vi "replace cursor action stack.vi"(7 "stack action":T2, 8 "action list I":T1[](array[typedef]), 9 "cursor action":T1=enum."write", 11 "command stack In":T1[](array[typedef])) -> (1 "cursor action Out":T1=enum."write", 2 "stack is empty ?":bool, 3 "command stack Out":T1[](array[typedef]))   [LabVIEW 2018]
uses:
  stack action -- control.ctl
  cursor action.ctl
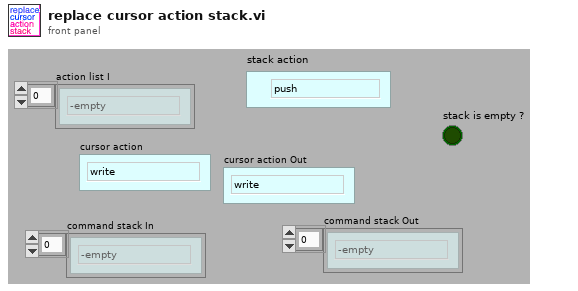
[diagram p1: front panel]
types:
  T1 = typedef "cursor action.ctl" = enum16{"range", "read", "write", "check", "zoom out", "smart zoom out", "zoom to aspect ratio 1", "zoom to win", "zoom out 20%", "zoom in 20%", "-empty", "smart zoom out&aspect", "move range left 20%", "move range right 20%", "move range up 20%", "move range down 20%", "zoom to X win", "zoom to Y win", "zoom out X", "zoom out Y", "zoom in X", "zoom in Y", "check plot scale"}
  T2 = typedef "stack action -- control.ctl" = enum16{"push", "pop", "check", "init"}
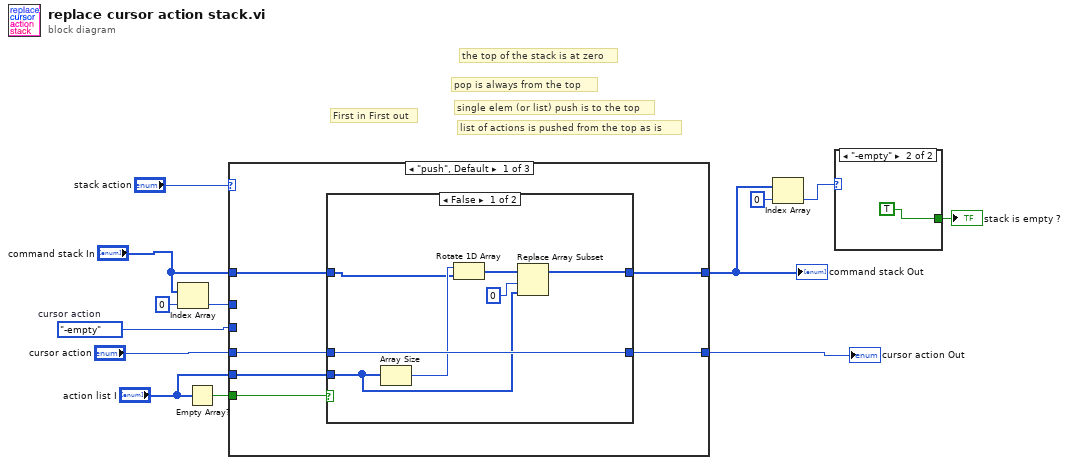
[diagram p0: block diagram]
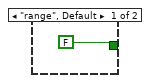
[diagram p2: hidden frame]
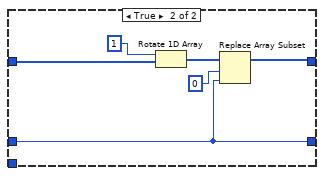
[diagram p3: hidden frame]
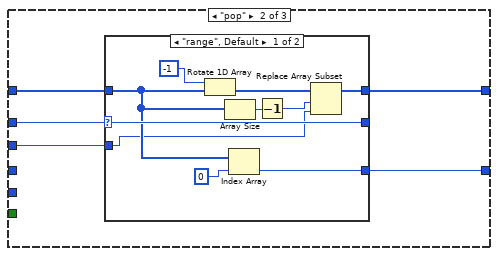
[diagram p4: hidden frame]
diagram:
  w6 = cursor_action."-empty"  # cursor action
  # "list of actions is pushed from the top as is"
  # "single elem (or list) push is to the top"
  # "pop is always from the top"
  # "First in First out"
  # "the top of the stack is at zero"
  n1 = Index Array(array="command stack In", index=0) -> (element=w10:T1)
  n2 = Empty Array?(array="action list I") -> (empty?=w12:bool)
  n3 = case shown="\"push\", Default" "stack action" {
    tunnel: [w19 w37 w51] -> w2
    tunnel: "command stack In" -> [w18 w36 w51]
    tunnel: w10 -> [_ w35 _]
    tunnel: [w14 w34 w52] -> w4
    tunnel: "cursor action" -> [w17 _ w52]
    tunnel: w12 -> [w16 _ _]
    tunnel: "action list I" -> [w15 _ _]
    tunnel: w6 -> [_ w33 _]
    frame "push", Default {
      n4 = case shown="False" w16 {
        tunnel: [w20 w27] -> w19
        tunnel: w18 -> [w24 w29]
        tunnel: w17 -> [w26 w30]
        tunnel: w15 -> [w21 _]
        tunnel: [w26 w30] -> w14
        frame False {
          n5 = Array Size(array=w21) -> (size(s)=w25:i32)
          n6 = Rotate 1D Array(1:w24, 2:w25) -> (0:w23:T1[])
          n7 = Replace Array Subset(array=w23, new element=w21, index=0) -> (w20:T1[])
        }
        frame True {
          n8 = Rotate 1D Array(1:w29, 2:1) -> (0:w32:T1[])
          n9 = Replace Array Subset(array=w32, new element=w30, index=0) -> (w27:T1[])
        }
      }
    }
    frame "pop" {
      n10 = case shown="\"range\", Default" w35 {
        selector: w35 -> [w45 w49]
        tunnel: [w41 w50] -> w37
        tunnel: w36 -> [w42 w50]
        tunnel: [w46 w48] -> w34
        tunnel: [w45 w49] -> _
        tunnel: w33 -> [w38 w48]
        frame "range", Default {
          n11 = Rotate 1D Array(1:w42, 2:-1) -> (0:w40:T1[])
          n12 = Array Size(array=w42) -> (size(s)=w43:i32)
          n13 = Index Array(array=w42, index=0) -> (element=w46:T1)
          n14 = Decrement(x=w43) -> (x-1=w39:i32)
          n15 = Replace Array Subset(array=w40, new element=w38, index=w39) -> (w41:T1[])
        }
        frame "-empty" {
        }
      }
    }
    frame "check" {
    }
  }
  "cursor action Out" <- w4
  "command stack Out" <- w2
  n16 = Index Array(array=w2, index=0) -> (element=w8:T1)
  n17 = case shown="\"-empty\"" w8 {
    tunnel: [FALSE TRUE] -> w7
    frame "range", Default {
    }
    frame "-empty" {
    }
  }
  "stack is empty ?" <- w7
